vi "main_Gesture data collection and signal processing.vi"() -> ()   [LabVIEW 2020]
uses:
  <vilib>/Analysis/3filter.llb/Filter Passband Type.ctl
  <vilib>/Analysis/3filter.llb/Butterworth Filter (DBL).vi
  <vilib>/express/express analysis/Spectral/Block/exnSpectralBlock spectral measurements power poly.vi
  <vilib>/express/express analysis/Spectral/Block/exnSpectralBlock spectral measurements power DDT.vi
  <vilib>/Utility/file.llb/Write Delimited Spreadsheet (DBL).vi
  <vilib>/express/express analysis/Spectral/XNode/ExpressSpectralMeasurementsBlockNode.xnode
  <vilib>/Analysis/NI_AALBase.lvlib
  <vilib>/Analysis/NI_AALPro.lvlib
  <vilib>/Analysis/NI_AAL_SigProc.lvlib
panel:
  out "XY Graph 4":cluster{"Y":dbl[], "Y":dbl[]}[](graph) caption="ML_集成树"
  out "XY Graph 3":cluster{"Y":dbl[], "Y":dbl[]}[](graph) caption="XY图"
  out "通道1":dynamicdata(graph)
  out "XY Graph 2":cluster{"Y":dbl[], "Y":dbl[]}[](graph) caption="ML_集成树"
  in  "训练——位置":dbl
  out "数值":dbl
  out "采样点 2":dbl
  out "采样点":dbl
  out "XY Graph":cluster{"Y":dbl[], "Y":dbl[]}[](graph) caption="XY图"
  out "ToF 2(cm)":dbl
  out "ToF 1(cm)":dbl
  out "有手势":bool
  out "最大值 1":dbl
  out "最大值2":dbl
  out "波形图 2":dbl[](graph)
  out "余数 2":dbl
  out "循环 2":dbl
  out "波形图":dbl[](graph)
  out "通道1_去环境噪声":dbl[](graph)
  out "通道2_去环境+滤波":dbl[](graph)
  out "频谱2":dynamicdata(graph)
  out "通道1_滤波":dbl[](graph)
  out "通道2_滤波":dbl[](graph)
  out "激励信号":dynamicdata(graph)
  out "通道2":dynamicdata(graph)
  in  "停止":bool
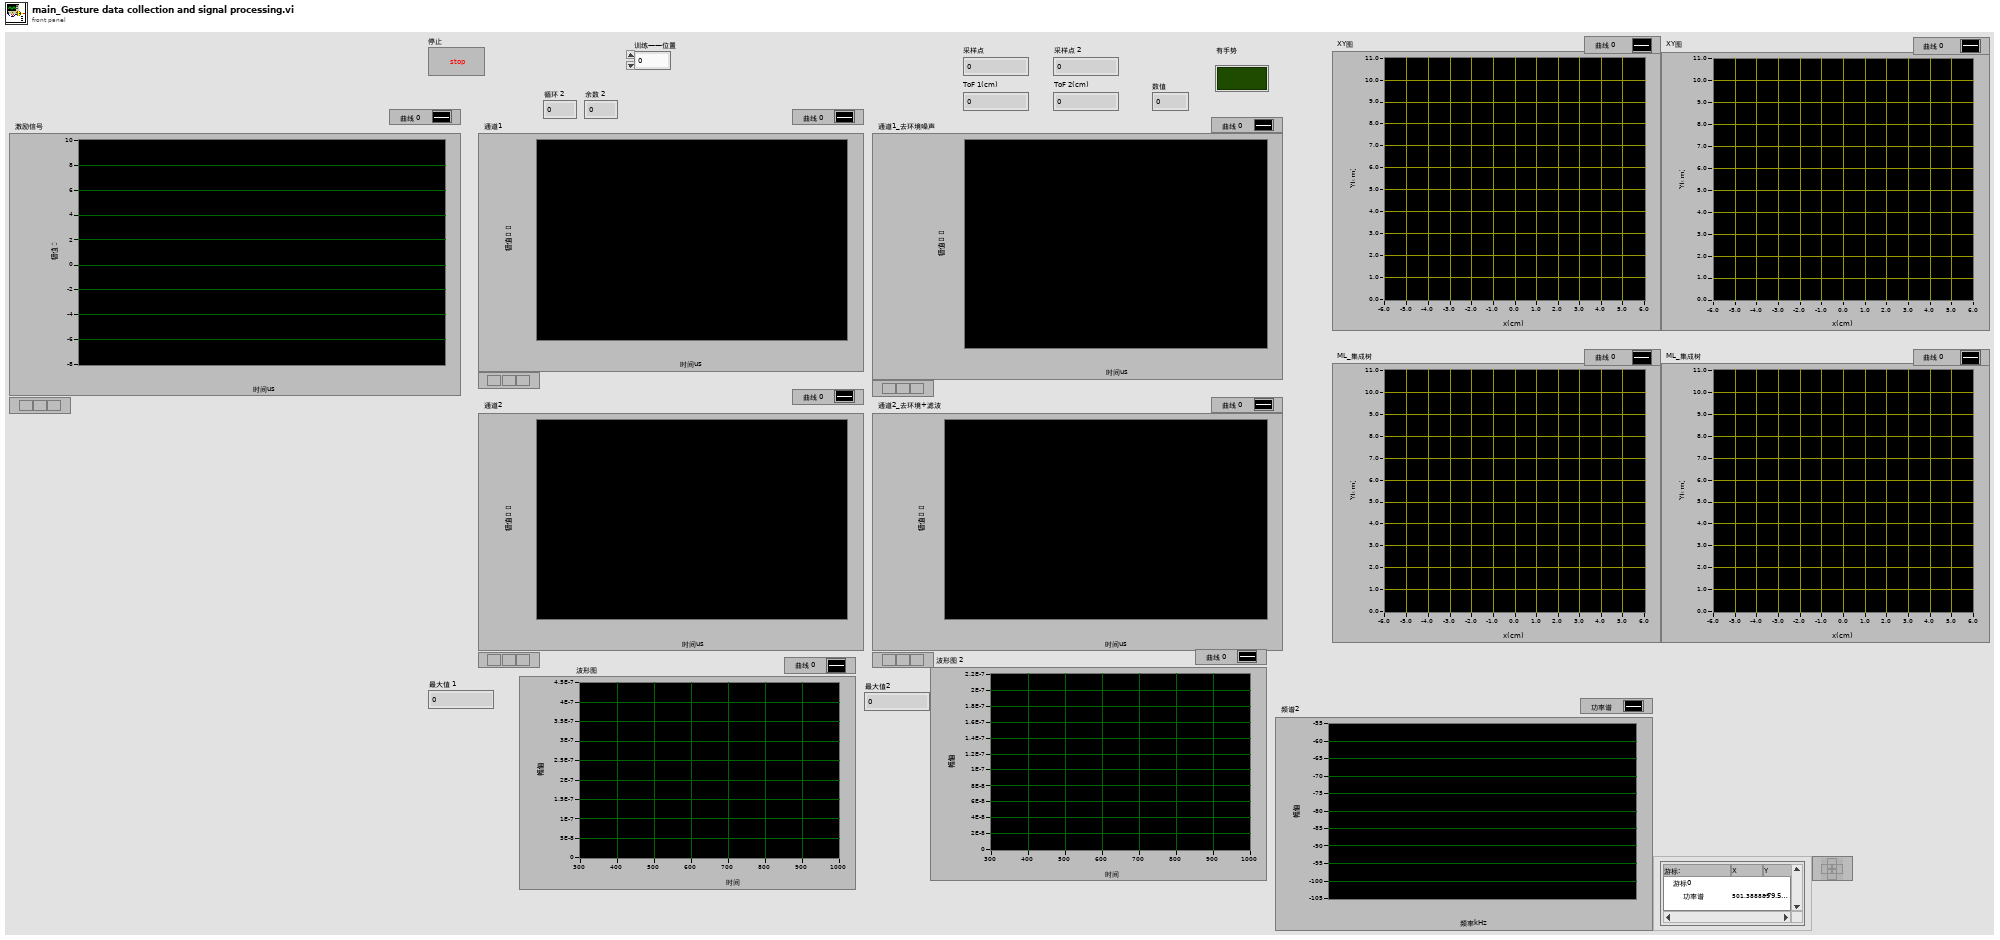
[diagram p1: front panel]
types:
  T1 = typedef "NI_AALBase.lvlib/Filter Passband Type.ctl" = enum32{"Lowpass", "Highpass", "Bandpass", "Bandstop"}
  T2 = cluster{"averaging mode":u16, "weighting mode":u16, "number of averages":u32}
  T3 = cluster{"dB On (F)":bool, "unwrap phase (F)":bool, "convert to degree (F)":bool}
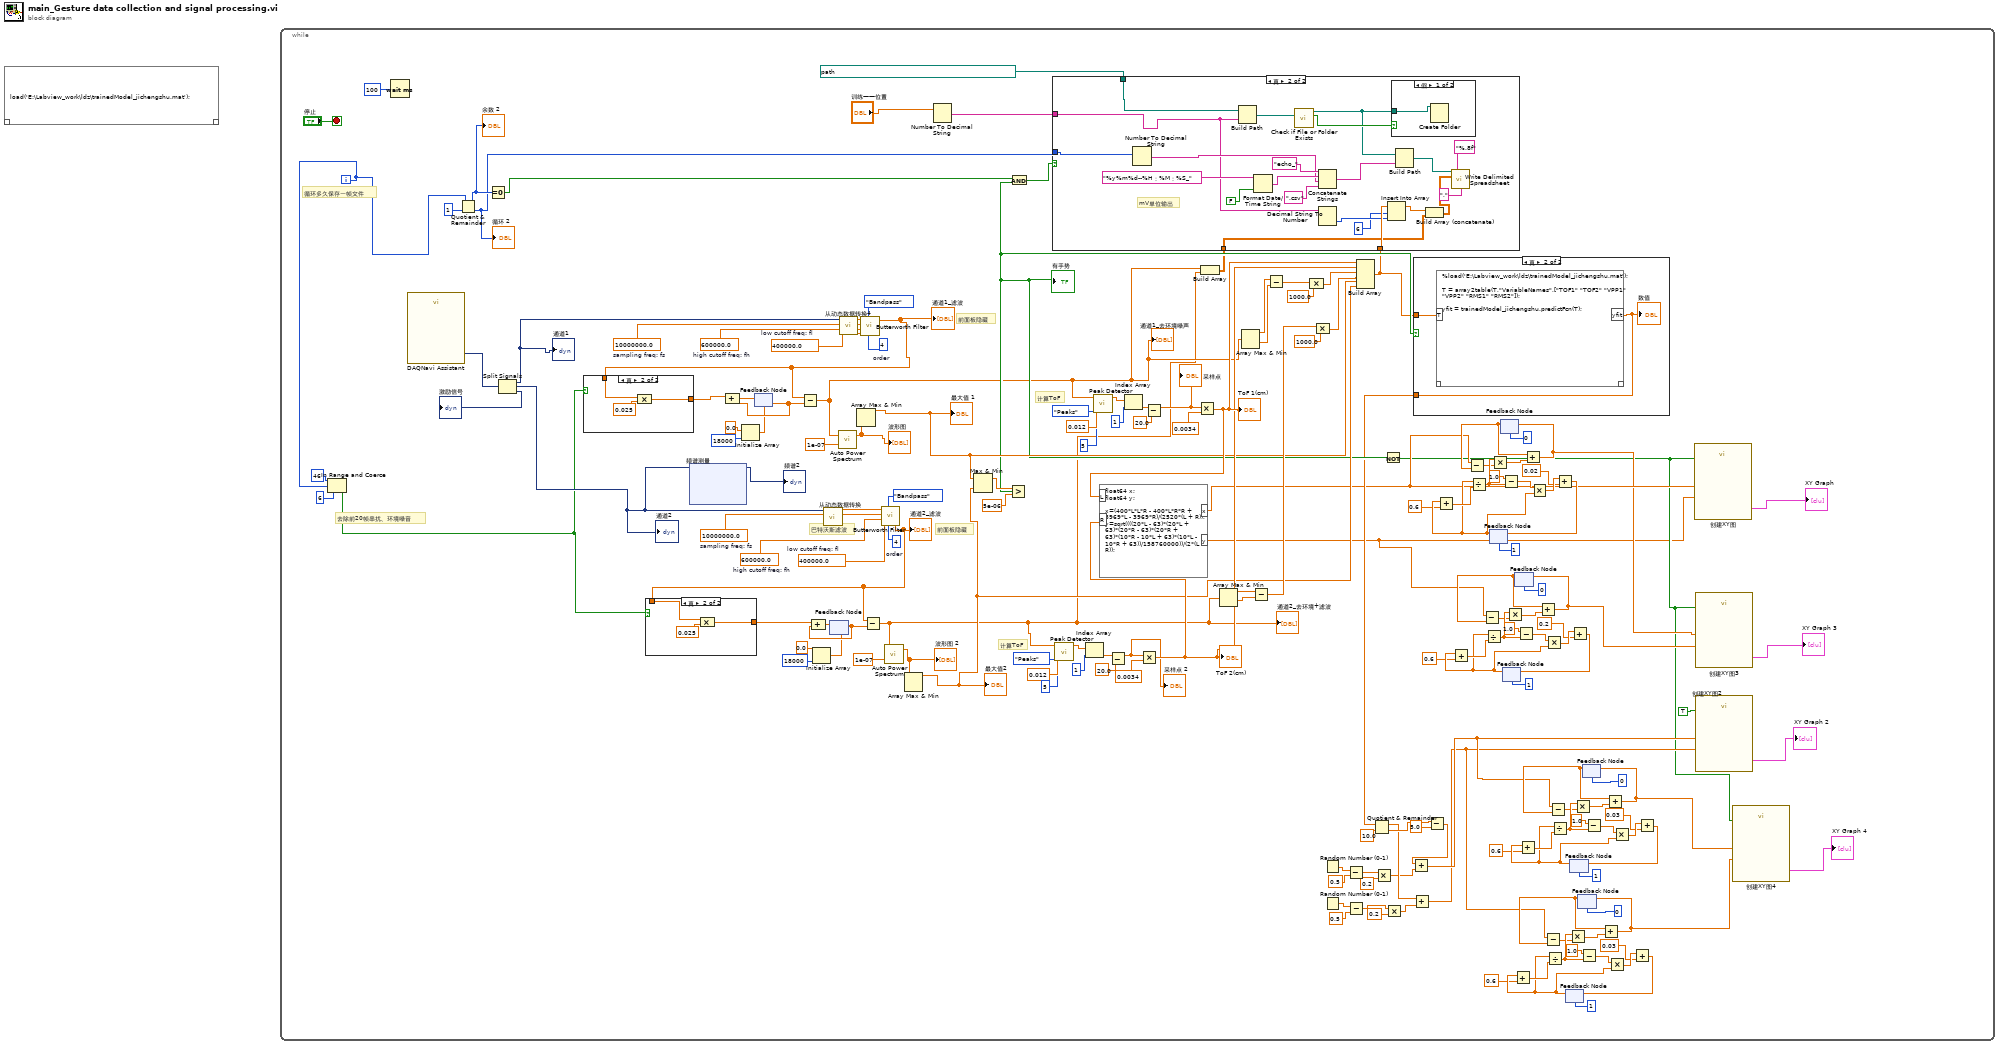
[diagram p0: block diagram]
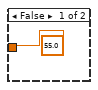
[diagram p2: hidden frame]
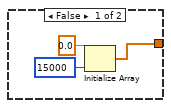
[diagram p5: hidden frame]
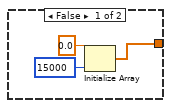
[diagram p6: hidden frame]
diagram:
  n1 = script code="load('E:\\Labview_work\\ldz\\trainedModel_jichengshu.mat');"() -> ()  [unwired: 1 in, 1 out]
  n2 = while {
    i -> [w139]
    stop <- "停止" stop-if-true
    w161 = 400000.0  # low cutoff freq: fl
    w165 = 600000.0  # high cutoff freq: fh
    w164 = 10000000.0  # sampling freq: fs
    w166 = 4  # order
    w172 = 400000.0  # low cutoff freq: fl
    w171 = 600000.0  # high cutoff freq: fh
    w170 = 10000000.0  # sampling freq: fs
    w173 = 4  # order
    # "计算ToF"
    # "计算ToF"
    # "前面板隐藏"
    # "前面板隐藏"
    # "去除前20帧串扰、环境噪音"
    # "循环多久保存一帧文件"
    # "巴特沃斯滤波"
    n3 = In Range and Coerce(upper limit=46 ("上限"), x=w139, lower limit=6 ("下限")) -> (In Range?=w143:bool)  [unwired: 1 out]
    n4 = Wait (ms)(milliseconds to wait=100) -> ()  [unwired: 1 out]
    n5 = call "DAQNavi Assistant"() -> ("data out(DDT)"=w159:dynamicdata)  [unwired: 6 in, 21 out]
    n6 = Quotient & Remainder(x=w139, y=1) -> (x-y*floor(x/y)=w141:i32, floor(x/y)=w140:i32)
    "循环 2" <- w140
    "余数 2" <- w141
    n7 = Equal To 0?(x=w141) -> (x = 0?=w130:bool)
    n8 = Split Signals(w159) -> (w78:dynamicdata, w160:dynamicdata, →"激励信号":dynamicdata)  [unwired: 3 in]
    "通道2" <- w160
    "通道1" <- w78
    n9 = xnode "频谱测量"("信号"=w160) -> ("功率谱"=→"频谱2":dynamicdata)  [unwired: 1 in, 1 out]
    n10 = Initialize Array(0.0 ("元素"), 18000 ("维数大小")) -> (w147:dbl[])
    n11 = feedback #1(w147) -> (w149:dbl[])
    n12 = Initialize Array(0.0 ("元素"), 18000 ("维数大小")) -> (w155:dbl[])
    n13 = call "从动态数据转换"("Dynamic Data Type"=w160) -> ("Array"=w168:dbl[])  [unwired: 3 in]
    n14 = feedback #2(w155) -> (w156:dbl[])
    n15 = call "从动态数据转换4"("Dynamic Data Type"=w78) -> ("Array"=w162:dbl[])  [unwired: 3 in]
    n16 = call-poly <vilib>:"Butterworth Filter.vi"("order"=w166, "filter type"=Filter_Passband_Type."Bandpass", "low cutoff freq: fl"=w161, "high cutoff freq: fh"=w165, "sampling freq: fs"=w164, "X"=w162) -> ("Filtered X"=w77:dbl[])  [unwired: 2 in, 1 out]
    "通道1_滤波" <- w77
    n17 = case shown="真" w143 {
      tunnel: w77 -> [_ w204]
      tunnel: [w201 w206] -> w151
      frame False {
        n18 = Initialize Array(0.0 ("元素"), 15000 ("维数大小")) -> (w201:dbl[])
      }
      frame True {
        n19 = Compound Arithmetic op=MULTIPLY(w204, 0.025) -> (w206:dbl[])
      }
    }
    n20 = Compound Arithmetic op=ADD(w151, w149) -> (w150:dbl[])
    n21 = feedback-in #1(w150) -> ()
    n22 = Subtract(x=w77, y=w149) -> (x-y=w3:dbl[])
    "通道1_去环境噪声" <- w3
    n23 = call <vilib>:"Auto Power Spectrum.vi"("dt"=1e-07, "Signal (V)"=w3) -> ("Power Spectrum (V^2 rms)"=w133:dbl[])  [unwired: 1 out]
    "波形图" <- w133
    n24 = Array Max & Min(array=w133) -> (max value=w102:dbl)  [unwired: 3 out]
    "最大值 1" <- w102
    n25 = call-poly <vilib>:"Butterworth Filter.vi"("order"=w173, "filter type"=Filter_Passband_Type."Bandpass", "low cutoff freq: fl"=w172, "high cutoff freq: fh"=w171, "sampling freq: fs"=w170, "X"=w168) -> ("Filtered X"=w152:dbl[])  [unwired: 2 in, 1 out]
    "通道2_滤波" <- w152
    n26 = case shown="真" w143 {
      tunnel: w152 -> [_ w212]
      tunnel: [w207 w211] -> w158
      frame False {
        n27 = Initialize Array(0.0 ("元素"), 15000 ("维数大小")) -> (w207:dbl[])
      }
      frame True {
        n28 = Compound Arithmetic op=MULTIPLY(w212, 0.025) -> (w211:dbl[])
      }
    }
    n29 = Compound Arithmetic op=ADD(w158, w156) -> (w157:dbl[])
    n30 = feedback-in #2(w157) -> ()
    n31 = Subtract(x=w152, y=w156) -> (x-y=w2:dbl[])
    "通道2_去环境+滤波" <- w2
    n32 = call <vilib>:"Auto Power Spectrum.vi"("dt"=1e-07, "Signal (V)"=w2) -> ("Power Spectrum (V^2 rms)"=w134:dbl[])  [unwired: 1 out]
    "波形图 2" <- w134
    n33 = Array Max & Min(array=w134) -> (max value=w101:dbl)  [unwired: 3 out]
    "最大值2" <- w101
    n34 = Number To Decimal String(number="训练——位置") -> (decimal integer string=w97:string)  [unwired: 1 in]
    n35 = Max & Min(x=w102, y=w101) -> (max(x,y)=w132:dbl)  [unwired: 1 out]
    n36 = Greater?(x=w132, y=5e-06) -> (0:w100:bool)
    "有手势" <- w100
    n37 = And(x=w130, y=w100) -> (x .and. y?=w129:bool)
    n38 = call <vilib>:"Peak Detector.vi"("peaks/valleys"=enum32{"Peaks", "Valleys"}."Peaks", "width"=5, "threshold"=0.012, "X"=w2) -> ("Locations"=w120:dbl[])  [unwired: 3 in, 4 out]
    n39 = Index Array(array=w120, index=1 ("索引")) -> (element=w73:dbl)
    n40 = call <vilib>:"Peak Detector.vi"("peaks/valleys"=enum32{"Peaks", "Valleys"}."Peaks", "width"=5, "threshold"=0.012, "X"=w3) -> ("Locations"=w125:dbl[])  [unwired: 3 in, 4 out]
    n41 = Subtract(x=w73, y=20.0) -> (x-y=w74:dbl)
    "采样点 2" <- w74
    n42 = Index Array(array=w125, index=1 ("索引")) -> (element=w118:dbl)
    n43 = Multiply(x=w74, y=0.0034) -> (x*y=w113:dbl)
    "ToF 2(cm)" <- w113
    n44 = Subtract(x=w118, y=20.0) -> (x-y=w76:dbl)
    "采样点" <- w76
    n45 = Multiply(x=w76, y=0.0034) -> (x*y=w114:dbl)
    "ToF 1(cm)" <- w114
    n46 = formula code="float64 x;\nfloat64 y; \n\nx=(400*L*L*R - 400*L*R*R + 3969*L - 3969*R)/(2520*(L + R));\ny=sqrt((((20*L - 63)*(20*L + 63)*(20*R - 63)*(20*R + 63)*(10*R - 10*L + 63)*(10*L - 10*R + 63))/158760000))/(2*(L + R));"("L"=w114, "R"=w113) -> ("x"=w57:dbl, "y"=w4:dbl)
    n47 = Build Array(w3, w2) -> (w1:dbl[][])
    n48 = Array Max & Min(array=w2) -> (max value=w105:dbl, min value=w104:dbl)  [unwired: 2 out]
    n49 = Array Max & Min(array=w3) -> (max value=w109:dbl, min value=w108:dbl)  [unwired: 2 out]
    n50 = Subtract(x=w105, y=w104) -> (x-y=w106:dbl)
    n51 = Subtract(x=w109, y=w108) -> (x-y=w107:dbl)
    n52 = Compound Arithmetic op=MULTIPLY(w107, 1000.0) -> (w111:dbl)
    n53 = Compound Arithmetic op=MULTIPLY(w106, 1000.0) -> (w103:dbl)
    n54 = Random Number (0-1)() -> (number: 0 to 1=w90:dbl)
    n55 = Random Number (0-1)() -> (number: 0 to 1=w87:dbl)
    n56 = Subtract(x=w90, y=0.5) -> (x-y=w84:dbl)
    n57 = Subtract(x=w87, y=0.5) -> (x-y=w79:dbl)
    n58 = Build Array(w114, w113, w111, w103, w102, w101) -> (w99:dbl[])
    n59 = case shown="真" w129 {
      tunnel: w140 -> [_ w190]
      tunnel: path "E:/Labview_work/ldz/数据/12.6/test" ("路径") -> [_ w187]
      tunnel: w99 -> [_ w185]
      tunnel: w97 -> [_ w181]
      tunnel: w1 -> [_ w180]
      frame False {
      }
      frame True {
        # "mV单位输出"
        n60 = Number To Decimal String(number=w190) -> (decimal integer string=w189:string)  [unwired: 1 in]
        n61 = Build Path(base path=w187, name or relative path=w181) -> (appended path=w194:path)
        n62 = Format Date/Time String ("格式化日期/时间字符串")(time format string (%c)="%y%m%d--%H：%M：%S_", UTC format=FALSE) -> (date/time string=w196:string)  [unwired: 1 in]
        n63 = call <vilib>:"Check if File or Folder Exists.vi"("path"=w194) -> ("file or folder exists?"=w193:bool, "dup path"=w182:path)  [unwired: 8 in, 1 out]
        n64 = Concatenate Strings("echo_" ("字符串"), w196, w189, ".csv" ("字符串")) -> (w198:string)
        n65 = Decimal String To Number(string=w181) -> (number=w184:i32)  [unwired: 2 in, 1 out]
        n66 = Insert Into Array(array=w185, index=6 ("索引"), new element=w184) -> (w179:dbl[])
        n67 = case shown="假" w193 {
          tunnel: w182 -> [w200 _]
          frame False {
            n68 = Create Folder(path (use dialog)=w200) -> ()  [unwired: 2 in, 3 out]
          }
          frame True {
          }
        }
        n69 = Build Path(base path=w182, name or relative path=w198) -> (appended path=w197:path)
        n70 = Build Array (concatenate)(w179, w180) -> (w178:dbl[][])
        n71 = call-poly <vilib>:"Write Delimited Spreadsheet.vi"("file path (dialog if empty)"=w197, "format (%.3f)"="%.8f", "2D data"=w178, "delimiter (\\t)"="," ("delimiter (\\t)")) -> ()  [unwired: 10 in, 2 out]
      }
    }
    n72 = Multiply(x=w84, y=0.2) -> (x*y=w83:dbl)
    n73 = Not(x=w100) -> (.not. x?=w5:bool)
    n74 = Multiply(x=w79, y=0.2) -> (x*y=w80:dbl)
    n75 = case shown="真" w100 {
      tunnel: w99 -> [_ w177]
      tunnel: [55.0 w176] -> w95
      frame False {
      }
      frame True {
        n76 = script code="%load('E:\\Labview_work\\ldz\\trainedModel_jichengshu.mat');\n\nT = array2table(T,\"VariableNames\",[\"TOF1\" \"TOF2\" \"VPP1\" \"VPP2\" \"RMS1\" \"RMS2\"]);\n\nyfit = trainedModel_jichengshu.predictFcn(T);" ("脚本节点")("T"=w177) -> ("yfit"=w176:dbl)  [unwired: 1 in, 1 out]
        "数值" <- w176
      }
    }
    n77 = Quotient & Remainder(x=w95, y=10.0) -> (x-y*floor(x/y)=w85:dbl, floor(x/y)=w93:dbl)
    n78 = Add(x=w85, y=w80) -> (x+y=w7:dbl)
    n79 = Subtract(x=w93, y=5.0) -> (x-y=w88:dbl)
    n80 = Add(x=w88, y=w83) -> (x+y=w23:dbl)
    n81 = feedback #3(1) -> (w63:dbl)
    n82 = Add(x=w63, y=0.6) -> (x+y=w71:dbl)
    n83 = Divide(x=w63, y=w71) -> (x/y=w69:dbl)
    n84 = feedback #4(0) -> (w62:dbl)
    n85 = Subtract(x=w57, y=w62) -> (x-y=w68:dbl)
    n86 = Multiply(x=w69, y=w68) -> (x*y=w67:dbl)
    n87 = Subtract(x=1.0, y=w69) -> (x-y=w66:dbl)
    n88 = feedback #5(1) -> (w45:dbl)
    n89 = Add(x=w45, y=0.6) -> (x+y=w53:dbl)
    n90 = Divide(x=w45, y=w53) -> (x/y=w51:dbl)
    n91 = feedback #6(0) -> (w44:dbl)
    n92 = Subtract(x=w4, y=w44) -> (x-y=w50:dbl)
    n93 = Multiply(x=w51, y=w50) -> (x*y=w49:dbl)
    n94 = Subtract(x=1.0, y=w51) -> (x-y=w48:dbl)
    n95 = Add(x=w62, y=w67) -> (x+y=w56:dbl)
    n96 = feedback-in #4(w56) -> ()
    n97 = Multiply(x=w66, y=w63) -> (x*y=w65:dbl)
    n98 = Add(x=w44, y=w49) -> (x+y=w39:dbl)
    n99 = feedback-in #6(w39) -> ()
    n100 = Multiply(x=w48, y=w45) -> (x*y=w47:dbl)
    n101 = Add(x=w65, y=0.02) -> (x+y=w64:dbl)
    n102 = feedback-in #3(w64) -> ()
    n103 = feedback #7(1) -> (w13:dbl)
    n104 = Add(x=w13, y=0.6) -> (x+y=w21:dbl)
    n105 = Divide(x=w13, y=w21) -> (x/y=w19:dbl)
    n106 = feedback #8(1) -> (w30:dbl)
    n107 = Add(x=w30, y=0.6) -> (x+y=w38:dbl)
    n108 = Divide(x=w30, y=w38) -> (x/y=w36:dbl)
    n109 = Add(x=w47, y=0.2) -> (x+y=w46:dbl)
    n110 = feedback-in #5(w46) -> ()
    n111 = feedback #9(0) -> (w12:dbl)
    n112 = Subtract(x=w7, y=w12) -> (x-y=w18:dbl)
    n113 = Multiply(x=w19, y=w18) -> (x*y=w17:dbl)
    n114 = Subtract(x=1.0, y=w19) -> (x-y=w16:dbl)
    n115 = feedback #10(0) -> (w29:dbl)
    n116 = Subtract(x=w23, y=w29) -> (x-y=w35:dbl)
    n117 = Multiply(x=w36, y=w35) -> (x*y=w34:dbl)
    n118 = Subtract(x=1.0, y=w36) -> (x-y=w33:dbl)
    n119 = Add(x=w12, y=w17) -> (x+y=w6:dbl)
    n120 = feedback-in #9(w6) -> ()
    n121 = Add(x=w29, y=w34) -> (x+y=w22:dbl)
    n122 = feedback-in #10(w22) -> ()
    n123 = Multiply(x=w16, y=w13) -> (x*y=w15:dbl)
    n124 = Multiply(x=w33, y=w30) -> (x*y=w32:dbl)
    n125 = Add(x=w15, y=0.03) -> (x+y=w14:dbl)
    n126 = feedback-in #7(w14) -> ()
    n127 = Add(x=w32, y=0.03) -> (x+y=w31:dbl)
    n128 = feedback-in #8(w31) -> ()
    n129 = call "创建XY图"("Reset"=w5, "Y Input"=w4, "X Input"=w57) -> ("XY Graph"=→"XY Graph":cluster{"X":dbl[], "Y":dbl[]}[])  [unwired: 7 in, 1 out]
    n130 = call "创建XY图2"("Reset"=TRUE, "Y Input"=w7, "X Input"=w23) -> ("XY Graph"=→"XY Graph 2":cluster{"X":dbl[], "Y":dbl[]}[])  [unwired: 7 in, 1 out]
    n131 = call "创建XY图3"("Reset"=w5, "Y Input"=w39, "X Input"=w56) -> ("XY Graph"=→"XY Graph 3":cluster{"X":dbl[], "Y":dbl[]}[])  [unwired: 7 in, 1 out]
    n132 = call "创建XY图4"("Reset"=w5, "Y Input"=w6, "X Input"=w22) -> ("XY Graph"=→"XY Graph 4":cluster{"X":dbl[], "Y":dbl[]}[])  [unwired: 7 in, 1 out]
  }
